vi "Timing Message Loop.vi"(8 "error in (no error)":errorcluster, 10 "Timers":T1, 11 "Message Queues":T2) -> (0 "error out":errorcluster)   [LabVIEW 2017, in "Message Queue.lvlib"]
uses:
  Message Queue.lvlib
  All Message Queues.ctl
  Message Cluster.ctl
  Acquisition/Acquisition State.ctl
  controls/ExitGlobal.vi
  Enqueue Message (Single).vi
  <vilib>/Utility/error.llb/Error Cluster From Error Code.vi
  <vilib>/ErrorRing/Error Ring.xnode
  Acquisition/Acquisition.lvlib
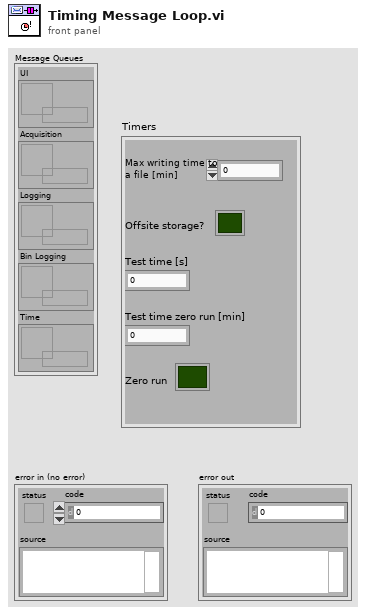
[diagram p1: front panel]
types:
  T1 = cluster{"Offsite storage?":bool, "Test time [s]":dbl, "Test time zero run [s] ":dbl, "Max writing time to a file [min]":dbl, "Zero run":bool}
  T2 = typedef "Message Queue.lvlib/All Message Queues.ctl" = cluster{"UI":refnum<queue>, "Acquisition":refnum<queue>, "Logging":refnum<queue>, "Bin Logging":refnum<queue>, "Time":refnum<queue>}
  T3 = typedef "Acquisition.lvlib/Acquisition State.ctl" = enum16{"Idle", "Acquiring"}
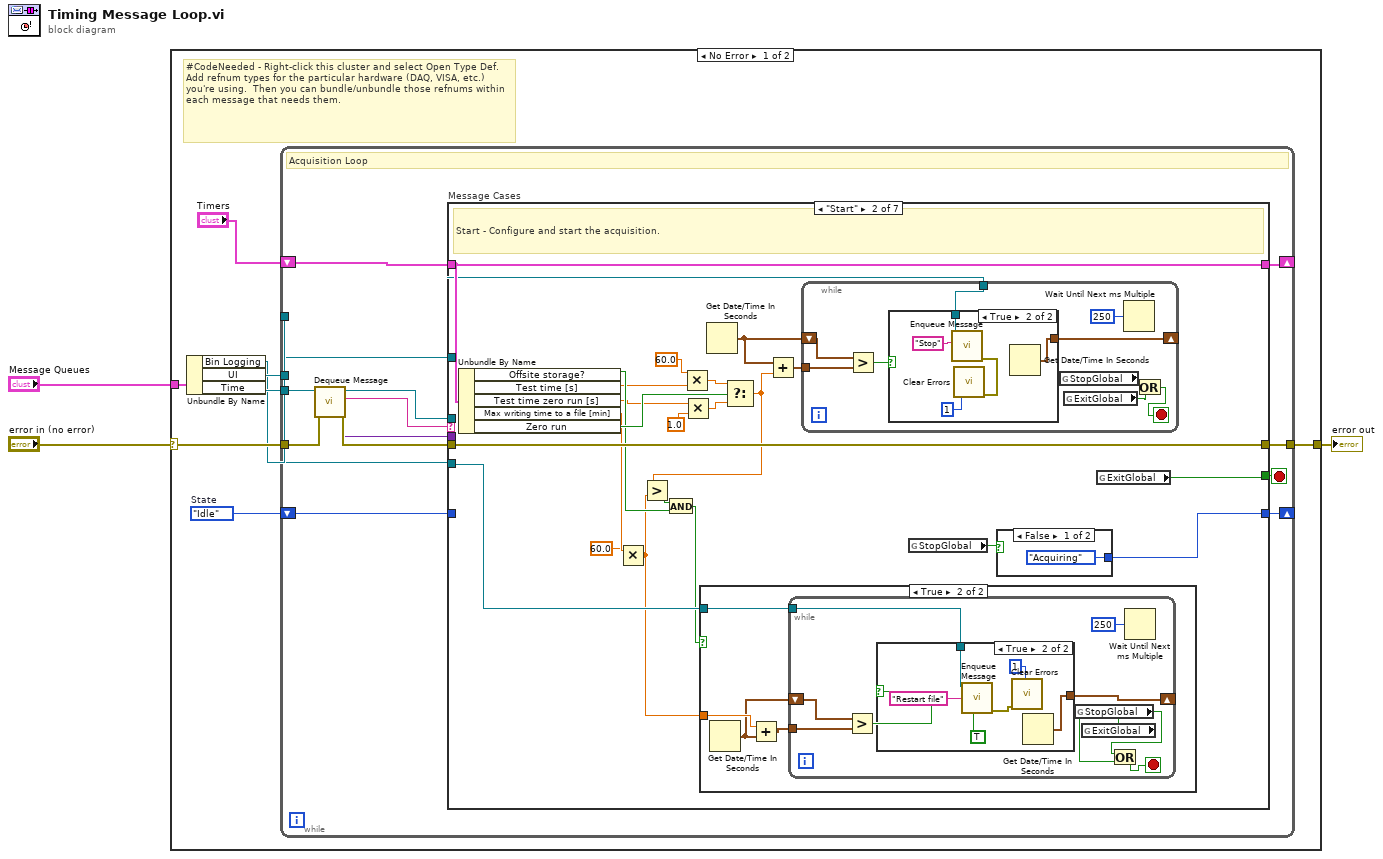
[diagram p0: block diagram]
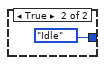
[diagram p3: hidden frame]
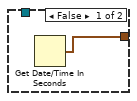
[diagram p4: hidden frame]
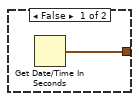
[diagram p6: hidden frame]
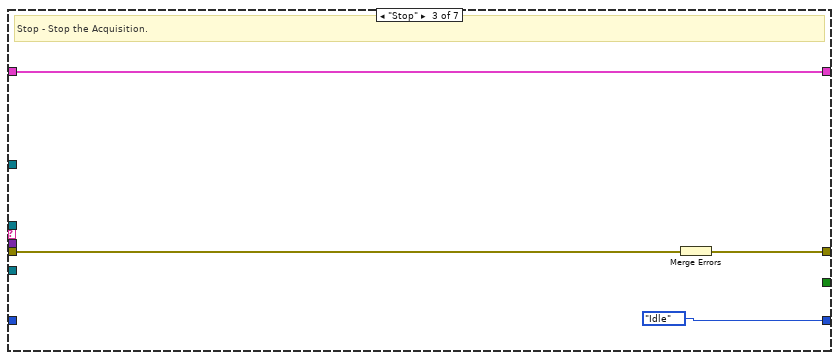
[diagram p7: hidden frame]
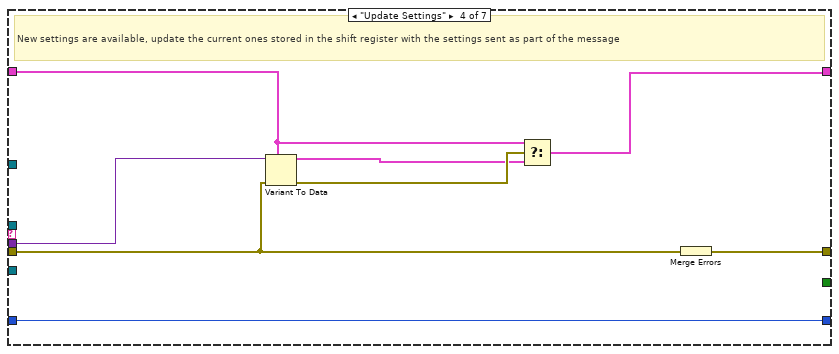
[diagram p8: hidden frame]
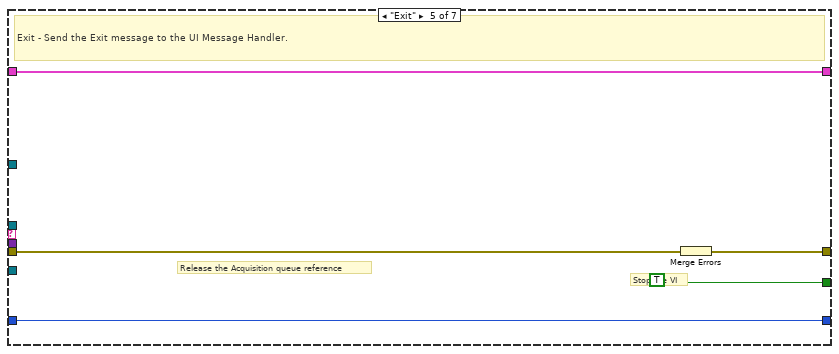
[diagram p9: hidden frame]
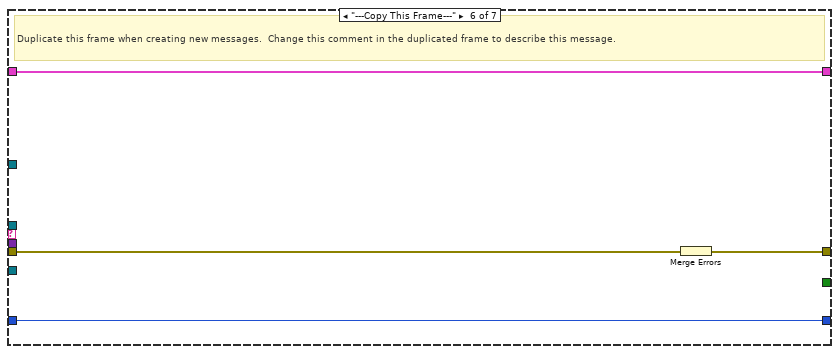
[diagram p10: hidden frame]
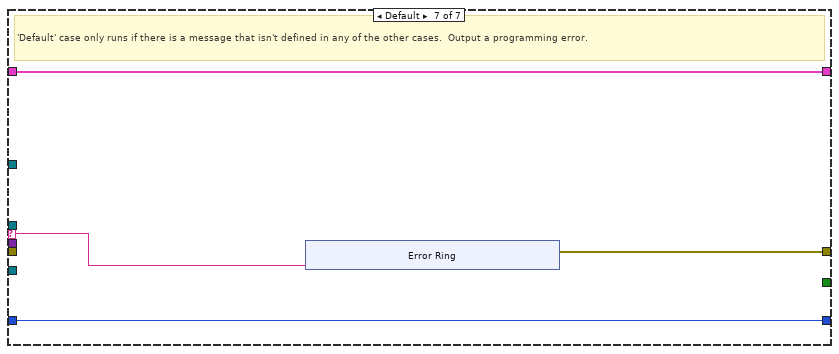
[diagram p11: hidden frame]
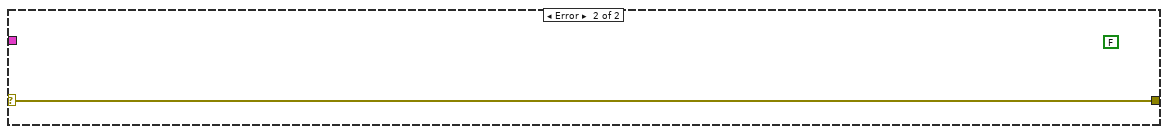
[diagram p12: hidden frame]
diagram:
  n1 = case shown="No Error" "error in (no error)" {
    selector: "error in (no error)" -> [w9 w121]
    tunnel: "Message Queues" -> [w11 _]
    tunnel: [w5 w121] -> w2
    frame No Error {
      w7 = Acquisition_State."Idle"  # State
      # "#CodeNeeded - Right-click this cluster and select Open Type Def.  Add refnum types for the particular hardware (DAQ, VISA, etc.) you're using.  Then you can bundle/unbundle those refnums within each message that needs them."
      n2 = Unbundle By Name(w11) -> ("Bin Logging"=w4:refnum<queue>, "UI"=w8:refnum<queue>, "Time"=w10:refnum<queue>)
      n3 = while {
        tunnel: w10 -> [w20]
        shift-right: [w24] -> _
        shift-left: "Timers" -> [w25]
        tunnel: w8 -> [w16]
        shift-right: [w18] -> _
        shift-left: w7 -> [w19]
        tunnel: w9 -> [w22]
        tunnel: [w15] -> w5
        tunnel: w4 -> [w14]
        stop <- w23 stop-if-true
        # "Acquisition Loop"
        n4 = call "Dequeue Message.vi"("error in (no error)"=w22, "Message Queue"=w20) -> ("error out"=w21:errorcluster, "Message Data"=w13:variant, "Message"=w12:string, "dup Message Queue"=w17:refnum<queue>)  [unwired: 6 in]
        n5 = case "Message Cases" shown="\"Start\"" w12 {
          selector: w12 -> [_ _ _ _ _ _ w110]
          tunnel: w17 -> [_ _ _ _ _ _ _]
          tunnel: w21 -> [w28 w51 w90 w96 w101 w109 _]
          tunnel: [w28 w51 w92 w100 w104 w107 w111] -> w15
          tunnel: w25 -> [w27 w49 w91 w93 w103 w108 w113]
          tunnel: [w27 w49 w91 w97 w103 w108 w113] -> w24
          tunnel: [_ w48 _ _ TRUE _ _] -> w23
          tunnel: w13 -> [_ _ _ w94 _ _ _]
          tunnel: w16 -> [_ w41 _ _ _ _ _]
          tunnel: w19 -> [w26 _ _ w95 w102 w106 w112]
          tunnel: [w26 w30 Acquisition_State."Idle" ("State") w95 w102 w106 w112] -> w18
          tunnel: w14 -> [_ w47 _ _ _ _ _]
          frame "Initialize" {
            # "Initialize  - Initialize is currently a no-op.  The hardware initialization takes place in the 'Start' message."
          }
          frame "Start" {
            # "Start - Configure and start the acquisition."
            n6 = Unbundle By Name(w49) -> ("Offsite storage?"=w42:bool, "Test time [s]"=w35:dbl, "Test time zero run [s]"=w39:dbl, "Max writing time to a file [min]"=w46:dbl, "Zero run"=w50:bool)
            n7 = Multiply(x=w46, y=60.0) -> (x*y=w31:dbl)
            n8 = Multiply(x=60.0 ("y"), y=w35) -> (x*y=w37:dbl)
            n9 = Multiply(x=w39, y=1.0) -> (x*y=w36:dbl)
            n10 = Get Date/Time In Seconds() -> (seconds since 1Jan1904=w32:timestamp)
            n11 = Select(t=w37, s=w50, f=w36) -> (s? t:f=w34:dbl)
            n12 = Greater?(x=w34, y=w31) -> (0:w43:bool)
            n13 = And(x=w43, y=w42) -> (x .and. y?=w44:bool)
            n14 = case shown="True" w44 {
              tunnel: w47 -> [_ w72]
              tunnel: w31 -> [_ w71]
              frame False {
              }
              frame True {
                n15 = Get Date/Time In Seconds() -> (seconds since 1Jan1904=w69:timestamp)
                n16 = Add(x=w71, y=w69) -> (x+y=w70:timestamp)
                n17 = while {
                  tunnel: w72 -> [w81]
                  tunnel: w70 -> [w79]
                  shift-right: [w76] -> _
                  shift-left: w69 -> [w78]
                  stop <- w73 stop-if-true
                  n18 = Greater?(x=w78, y=w79) -> (0:w77:bool)
                  n19 = case shown="True" w77 {
                    tunnel: w81 -> [_ w88]
                    tunnel: [w82 w83] -> w76
                    frame False {
                      n20 = Get Date/Time In Seconds() -> (seconds since 1Jan1904=w82:timestamp)
                    }
                    frame True {
                      n21 = call-poly "Enqueue Message.vi"("Priority Message? (F)"=TRUE, "Message"="Restart file" ("t"), "Message Queue"=w88) -> ("error out"=w87:errorcluster)  [unwired: 7 in, 1 out]
                      n22 = call <vilib>:"Clear Errors.vi"("error in (no error)"=w87, "specific error code to clear (0: all)"=1) -> ()  [unwired: 4 in, 2 out]
                      n23 = Get Date/Time In Seconds() -> (seconds since 1Jan1904=w83:timestamp)
                    }
                  }
                  n24 = global read "ExitGlobal.vi" "StopGlobal"() -> (w75:bool)
                  n25 = global read "ExitGlobal.vi" "ExitGlobal"() -> (w74:bool)
                  n26 = Or(x=w75, y=w74) -> (x .or. y?=w73:bool)
                  n27 = Wait Until Next ms Multiple(millisecond multiple=u32 250) -> ()  [unwired: 1 out]
                }
              }
            }
            n28 = Add(x=w32, y=w34) -> (x+y=w33:timestamp)
            n29 = while {
              tunnel: w41 -> [w62]
              tunnel: w33 -> [w60]
              shift-right: [w57] -> _
              shift-left: w32 -> [w58]
              stop <- w54 stop-if-true
              n30 = Greater?(x=w58, y=w60) -> (0:w59:bool)
              n31 = case shown="True" w59 {
                tunnel: w62 -> [_ w68]
                tunnel: [w63 w64] -> w57
                frame False {
                  n32 = Get Date/Time In Seconds() -> (seconds since 1Jan1904=w63:timestamp)
                }
                frame True {
                  n33 = call-poly "Enqueue Message.vi"("Message"="Stop" ("value in"), "Message Queue"=w68) -> ("error out"=w66:errorcluster)  [unwired: 8 in, 1 out]
                  n34 = call <vilib>:"Clear Errors.vi"("error in (no error)"=w66, "specific error code to clear (0: all)"=1) -> ()  [unwired: 4 in, 2 out]
                  n35 = Get Date/Time In Seconds() -> (seconds since 1Jan1904=w64:timestamp)
                }
              }
              n36 = global read "ExitGlobal.vi" "StopGlobal"() -> (w56:bool)
              n37 = global read "ExitGlobal.vi" "ExitGlobal"() -> (w55:bool)
              n38 = Wait Until Next ms Multiple(millisecond multiple=u32 250) -> ()  [unwired: 1 out]
              n39 = Or(x=w56, y=w55) -> (x .or. y?=w54:bool)
            }
            n40 = global read "ExitGlobal.vi" "StopGlobal"() -> (w29:bool)
            n41 = case shown="False" w29 {
              tunnel: [Acquisition_State."Acquiring" ("State") Acquisition_State."Idle" ("State")] -> w30
              frame False {
              }
              frame True {
              }
            }
            n42 = global read "ExitGlobal.vi" "ExitGlobal"() -> (w48:bool)
          }
          frame "Stop" {
            # "Stop - Stop the Acquisition."
            n43 = Merge Errors(w90) -> (w92:errorcluster)
          }
          frame "Update Settings" {
            # "New settings are available, update the current ones stored in the shift register with the settings sent as part of the message"
            n44 = Variant To Data(error in=w96, type=w93, Variant=w94) -> (data=w98:T1, error out=w99:errorcluster)
            n45 = Select(t=w93, s=w99, f=w98) -> (s? t:f=w97:T1)
            n46 = Merge Errors(w96) -> (w100:errorcluster)
          }
          frame "Exit" {
            # "Release the Acquisition queue reference"
            # "Stop the VI"
            # "Exit - Send the Exit message to the UI Message Handler."
            n47 = Merge Errors(w101) -> (w104:errorcluster)
          }
          frame "---Copy This Frame---" {
            # "Duplicate this frame when creating new messages.  Change this comment in the duplicated frame to describe this message."
            n48 = Merge Errors(w109) -> (w107:errorcluster)
          }
          frame Default {
            # "'Default' case only runs if there is a message that isn't defined in any of the other cases.  Output a programming error."
            n49 = xnode "Error Ring"("parameter 0"=w110) -> ("error out"=w111:errorcluster)
          }
        }
      }
    }
    frame Error {
      (unwired) FALSE ("Running")
    }
  }
  "error out" <- w2
